vi "Object orientation + stepper control with controlled grab.vi"() -> ()   [LabVIEW 2018]
uses:
  <vilib>/userdefined/High Color/IMAQdx.ctl
  Underlying VI's/Modified webcam FGV/Webcam AE.ctl
  Underlying VI's/I2C Master VI/I2C_MASTER_WRITE_NEW Type Def.ctl
panel:
  in  "Grab":bool
  in  "ENA":bool
  in  "Arduino mode":T1
  out "Corrected stepper":u8
  out "error out":errorcluster
  out "Error out":errorcluster
  in  "stop":bool
  out "Image":T2(plugin-control)
  out "Object Center Coordinates":cluster{"x":sgl, "y":sgl}
  out "Object detection cluster":T3
  in  "Mode":enum16{"Ball", "Soap", "Gel", "Pipe", "None"}(ring)
  # "Save me pls"
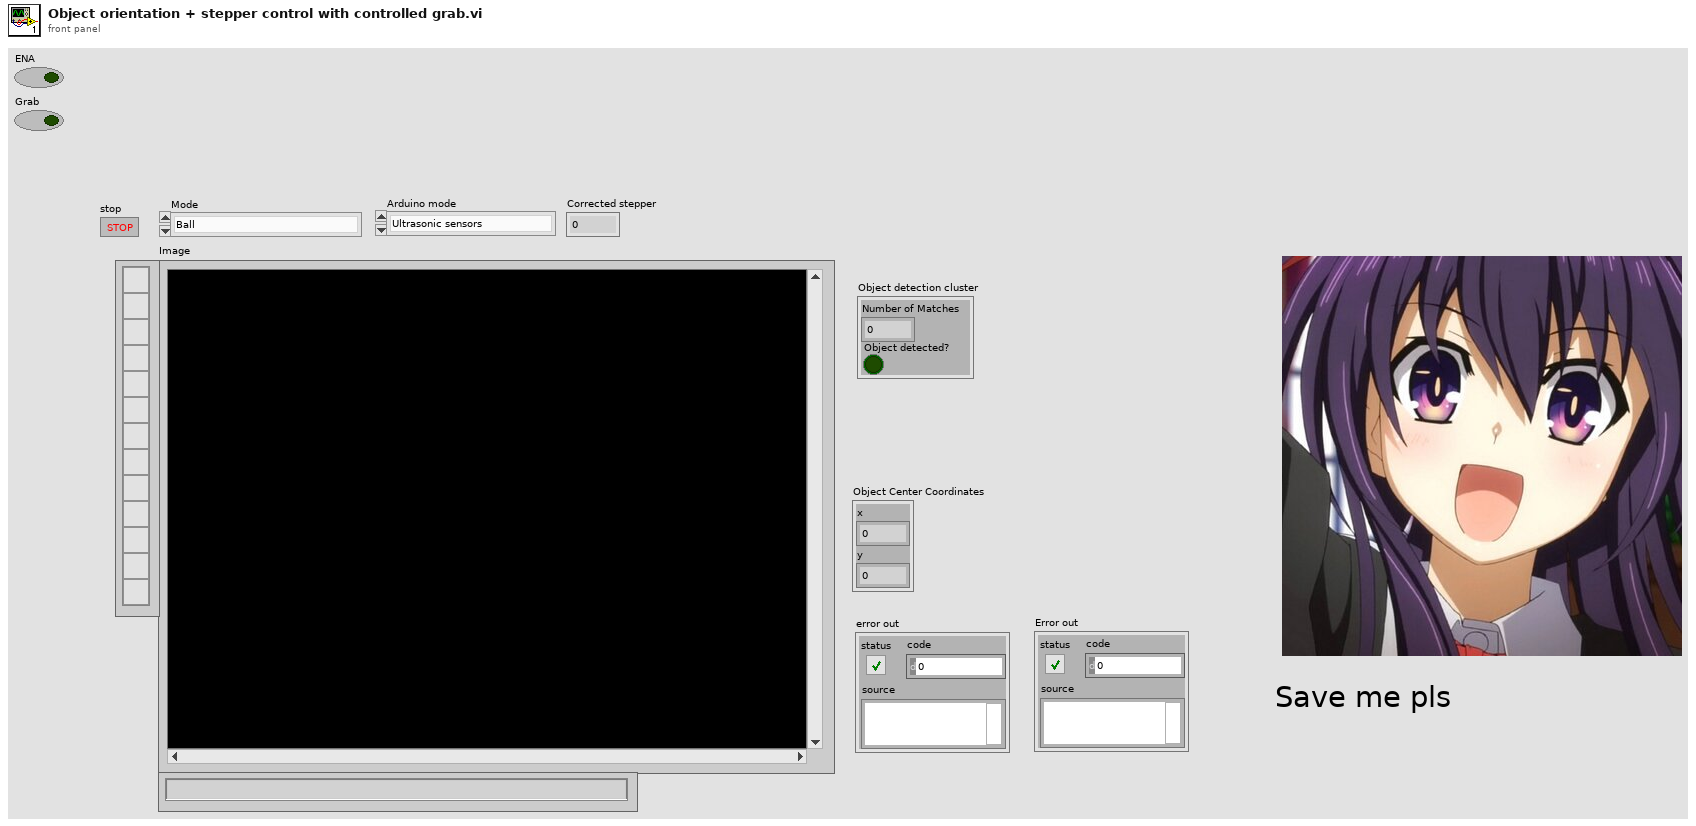
[diagram p1: front panel]
types:
  T1 = typedef "I2C_MASTER_WRITE_NEW Type Def.ctl" = enum16{"Ultrasonic sensors", "Stepper origin", "zStepper 13.3k", "zStepper 13k", "zStepper 12k", "zStepper 11k", "zStepper 10k", "zStepper 9k", "zStepper 8k", "zStepper 7k", "zStepper 6k", "zStepper 5k", "zStepper 4k", "zStepper 3k", "zStepper 2k", "zStepper 1k", "zStepper 900", "zStepper 800", "zStepper 700", "zStepper 600", "zStepper 500", "zStepper 400", "zStepper 300", "zStepper 200", "zStepper 100", "zStepper 0", "yStepper control", "Open Claw", "Close Claw", "Soft Reset"}
  T2 = typedef "IMAQ Image.ctl" = refnum<image>
  T3 = cluster{"Number of Matches":i32, "Object detected?":bool}
  T4 = typedef "Webcam AE.ctl" = enum16{"Initialize Camera", "Open Camera", "Continuous Acquisition", "Close Camera", "Retrieve Image", "Dispose Image Buffers"}
  T5 = typedef "Webcam AE.ctl" = enum16{"Initialize Camera", "Open Camera", "Continuous Acquisition", "Close Camera", "Retrieve Image", "Dispose Camera Image Buffer"}
  T6 = typedef "IMAQdx.ctl" = refnum<k21>
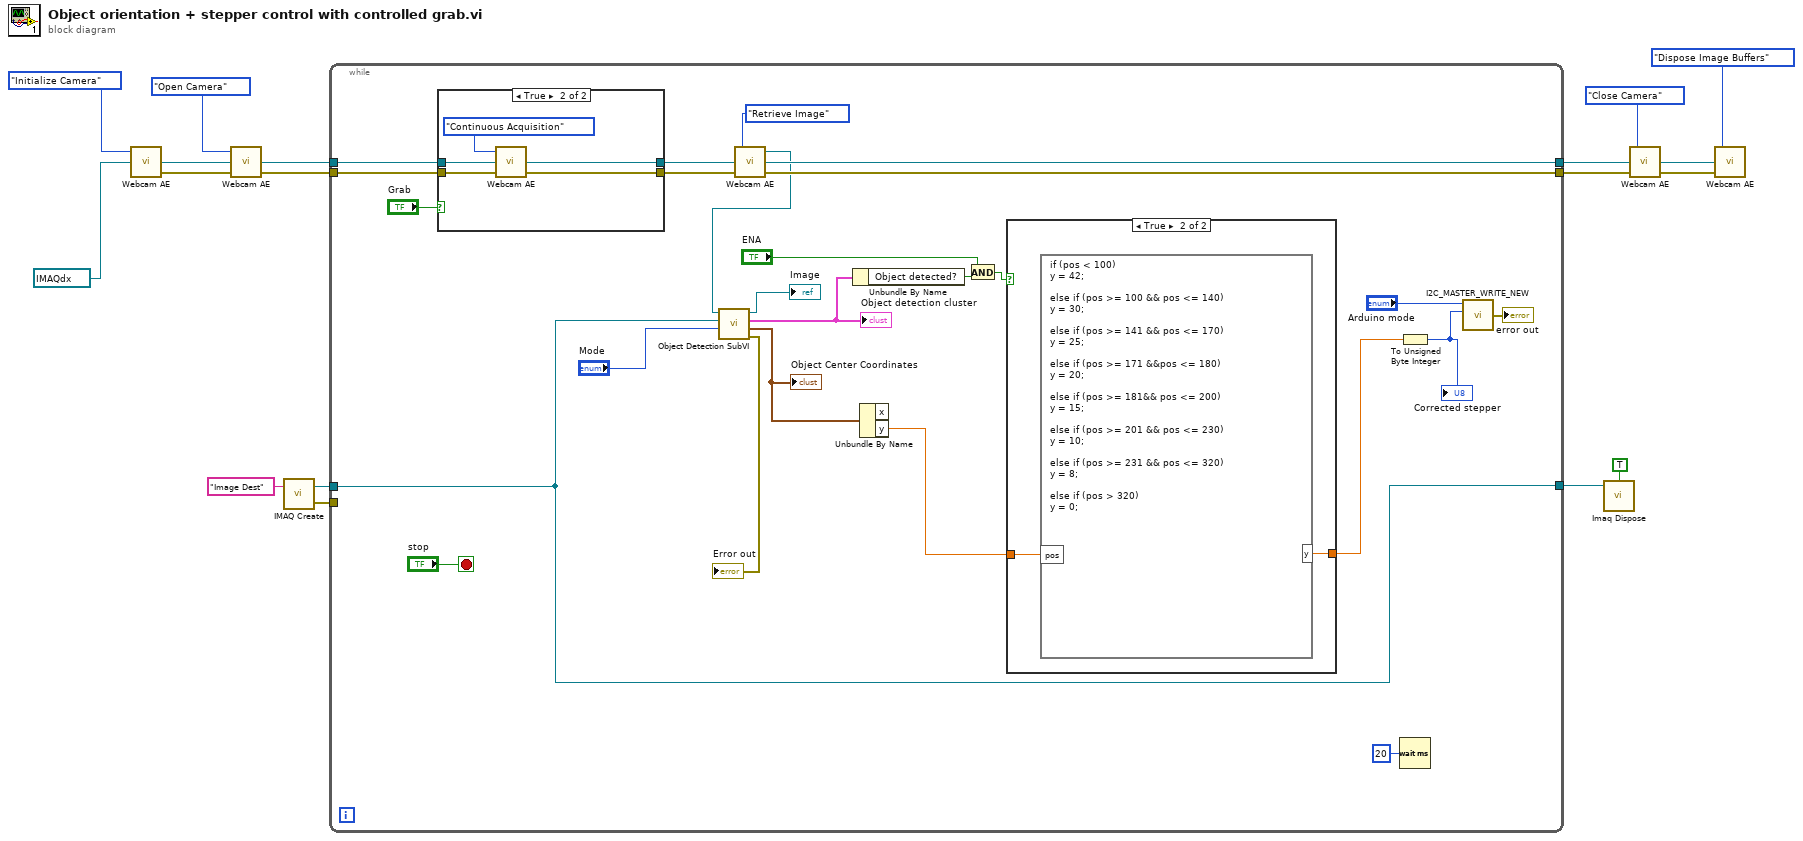
[diagram p0: block diagram]
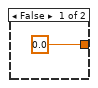
[diagram p3: hidden frame]
diagram:
  n1 = call "Webcam AE.vi"("Session In"=T6 "cam0", "Camera states"=Webcam_AE."Initialize Camera") -> ("error out"=w13:errorcluster, "Session Out"=w9:T6)  [unwired: 1 in, 1 out]
  n2 = call "Webcam AE.vi"("error in (no error)"=w13, "Session In"=w9, "Camera states"=Webcam_AE."Open Camera") -> ("error out"=w12:errorcluster, "Session Out"=w8:T6)  [unwired: 1 out]
  n3 = call "IMAQ Create"("Image Name"="Image Dest") -> ("New Image"=w18:T2, "error out"=w15:errorcluster)  [unwired: 4 in]
  n4 = while {
    tunnel: w18 -> [w39]
    tunnel: [w39] -> w16
    tunnel: w15 -> [_]
    tunnel: w12 -> [w27]
    tunnel: [w25] -> w11
    tunnel: w8 -> [w24]
    tunnel: [w22] -> w7
    stop <- "stop" stop-if-true
    n5 = case shown="True" "Grab" {
      tunnel: w27 -> [w44 w50]
      tunnel: [w44 w49] -> w26
      tunnel: w24 -> [w45 w48]
      tunnel: [w45 w47] -> w23
      frame False {
      }
      frame True {
        n6 = call "Webcam AE.vi"("error in (no error)"=w50, "Session In"=w48, "Camera states"=Webcam_AE."Continuous Acquisition") -> ("error out"=w49:errorcluster, "Session Out"=w47:T6)  [unwired: 1 out]
      }
    }
    n7 = call "Webcam AE.vi"("error in (no error)"=w26, "Session In"=w23, "Camera states"=Webcam_AE."Retrieve Image") -> ("error out"=w25:errorcluster, "Session Out"=w22:T6, "Image Out"=w19:T2)
    n8 = call "Object Detection SubVI.vi"("Mode"="Mode", "Image Dest"=w39, "Image in"=w19) -> ("Error out"=→"Error out":errorcluster, "Object Center Coordinates"=w37:cluster{"x":sgl, "y":sgl}, "Object detection cluster"=w31:T3, "Image Out"=→"Image":T2)  [unwired: 1 in]
    "Object detection cluster" <- w31
    "Object Center Coordinates" <- w37
    n9 = Unbundle By Name(w31) -> ("Object detected?"=w30:bool)
    n10 = Unbundle By Name(w37) -> ("y"=w33:sgl)  [unwired: 1 out]
    n11 = And(x="ENA", y=w30) -> (x .and. y?=w28:bool)
    n12 = case shown="True" w28 {
      tunnel: w33 -> [_ w53]
      tunnel: [0.0 ("y") w52] -> w32
      frame False {
      }
      frame True {
        n13 = formula code="if (pos < 100)\ny = 42;\n\nelse if (pos >= 100 && pos <= 140)\ny = 30;\n\nelse if (pos >= 141 && pos <= 170)\ny = 25;\n\nelse if (pos >= 171 &&pos <= 180) \ny = 20;\n\nelse if (pos >= 181&& pos <= 200)\ny = 15;\n\nelse if (pos >= 201 && pos <= 230)\ny = 10;\n\nelse if (pos >= 231 && pos <= 320)\ny = 8;\n\nelse if (pos > 320)\ny = 0;"("pos"=w53) -> ("y"=w52:dbl)
      }
    }
    n14 = To Unsigned Byte Integer(number=w32) -> (unsigned 8bit integer=w35:u8)
    "Corrected stepper" <- w35
    n15 = Wait (ms)(milliseconds to wait=u32 20) -> ()  [unwired: 1 out]
    n16 = call "I2C_MASTER_WRITE_NEW.vi"("y Stepper value"=w35, "Arduino mode"="Arduino mode") -> ("error out"=→"error out":errorcluster)  [unwired: 2 in]
  }
  n17 = call "Imaq Dispose"("All Images? (No)"=TRUE, "Image"=w16) -> ()  [unwired: 4 in, 1 out]
  n18 = call "Webcam AE.vi"("error in (no error)"=w11, "Session In"=w7, "Camera states"=Webcam_AE."Close Camera") -> ("error out"=w10:errorcluster, "Session Out"=w6:T6)  [unwired: 1 out]
  n19 = call "Webcam AE.vi"("error in (no error)"=w10, "Session In"=w6, "Camera states"=Webcam_AE."Dispose Image Buffers") -> ()  [unwired: 3 out]
